vi "Recipe Editor.vi"() -> ()   [LabVIEW 2015, in "Formation.lvclass"]
uses:
  Formation.lvclass
  Type Defs/Action Enum.ctl
  Type Defs/Direction Enum.ctl
  Type Defs/SB Type Defs.lvlib
panel:
  out "Recipe 2":T3(array[cluster])
  out "Recipe":T3(array[cluster])=[{"Options"=[]}, {"Options"=[]}, {"Options"=[{"X"=1, "Y"=0, "SignMatch"=0, "Action"=enum."Attack", "Direction"=enum."N", "Unit Idx"=252}, {"X"=1, "Y"=1, "SignMatch"=0, "Action"=enum."Wait", "Direction"=enum."E", "Unit Idx"=2}]}, {"Options"=[{"X"=1, "Y"=0, "SignMatch"=0, "Action"=enum."Attack", "Direction"=enum."N", "Unit Idx"=253}, {"X"=1, "Y"=1, "SignMatch"=0, "Action"=enum."Wait", "Direction"=enum."E", "Unit Idx"=3}]}, {"Options"=[]}, {"Options"=[]}, {"Options"=[]}, {"Options"=[{"X"=0, "Y"=0, "SignMatch"=0, "Action"=enum."Attack", "Direction"=enum."NW", "Unit Idx"=0}, {"X"=1, "Y"=0, "SignMatch"=0, "Action"=enum."Attack", "Direction"=enum."N", "Unit Idx"=1}, {"X"=0, "Y"=1, "SignMatch"=0, "Action"=enum."Attack", "Direction"=enum."W", "Unit Idx"=6}, {"X"=1, "Y"=1, "SignMatch"=1, "Action"=enum."Wait", "Direction"=enum."E", "Unit Idx"=7}]}, {"Options"=[{"X"=1, "Y"=0, "SignMatch"=0, "Action"=enum."Move", "Direction"=enum."N", "Unit Idx"=2}, {"X"=1, "Y"=1, "SignMatch"=1, "Action"=enum."Wait", "Direction"=enum."E", "Unit Idx"=8}]}, {"Options"=[{"X"=1, "Y"=0, "SignMatch"=0, "Action"=enum."Move", "Direction"=enum."N", "Unit Idx"=3}, {"X"=1, "Y"=1, "SignMatch"=1, "Action"=enum."Wait", "Direction"=enum."E", "Unit Idx"=9}]}, {"Options"=[{"X"=2, "Y"=0, "SignMatch"=0, "Action"=enum."Attack", "Direction"=enum."NE", "Unit Idx"=5}, {"X"=1, "Y"=0, "SignMatch"=0, "Action"=enum."Attack", "Direction"=enum."N", "Unit Idx"=4}, {"X"=2, "Y"=1, "SignMatch"=0, "Action"=enum."Attack", "Direction"=enum."E", "Unit Idx"=11}, {"X"=1, "Y"=1, "SignMatch"=1, "Action"=enum."Wait", "Direction"=enum."E", "Unit Idx"=10}]}, {"Options"=[]}, {"Options"=[{"X"=0, "Y"=1, "SignMatch"=0, "Action"=enum."Attack", "Direction"=enum."W", "Unit Idx"=11}, {"X"=1, "Y"=1, "SignMatch"=0, "Action"=enum."Wait", "Direction"=enum."E", "Unit Idx"=12}]}, {"Options"=[{"X"=0, "Y"=1, "SignMatch"=0, "Action"=enum."Move", "Direction"=enum."W", "Unit Idx"=12}, {"X"=1, "Y"=0, "SignMatch"=0, "Action"=enum."Move", "Direction"=enum."N", "Unit Idx"=7}, {"X"=1, "Y"=1, "SignMatch"=1, "Action"=enum."Wait", "Direction"=enum."E", "Unit Idx"=13}]}, {"Options"=[{"X"=2, "Y"=1, "SignMatch"=0, "Action"=enum."Replicate", "Direction"=enum."E", "Unit Idx"=15}, {"X"=1, "Y"=2, "SignMatch"=0, "Action"=enum."Replicate", "Direction"=enum."S", "Unit Idx"=20}, {"X"=1, "Y"=0, "SignMatch"=0, "Action"=enum."Replicate", "Direction"=enum."N", "Unit Idx"=8}, {"X"=0, "Y"=1, "SignMatch"=0, "Action"=enum."Replicate", "Direction"=enum."W", "Unit Idx"=13}, {"X"=1, "Y"=1, "SignMatch"=1, "Action"=enum."Wait", "Direction"=enum."E", "Unit Idx"=14}]}, {"Options"=[{"X"=1, "Y"=2, "SignMatch"=0, "Action"=enum."Replicate", "Direction"=enum."S", "Unit Idx"=21}, {"X"=1, "Y"=0, "SignMatch"=0, "Action"=enum."Replicate", "Direction"=enum."N", "Unit Idx"=9}, {"X"=2, "Y"=1, "SignMatch"=0, "Action"=enum."Replicate", "Direction"=enum."E", "Unit Idx"=16}, {"X"=1, "Y"=1, "SignMatch"=1, "Action"=enum."Wait", "Direction"=enum."E", "Unit Idx"=15}]}, {"Options"=[{"X"=2, "Y"=1, "SignMatch"=0, "Action"=enum."Move", "Direction"=enum."E", "Unit Idx"=17}, {"X"=1, "Y"=0, "SignMatch"=0, "Action"=enum."Move", "Direction"=enum."N", "Unit Idx"=10}, {"X"=1, "Y"=1, "SignMatch"=1, "Action"=enum."Wait", "Direction"=enum."E", "Unit Idx"=16}]}, {"Options"=[{"X"=2, "Y"=1, "SignMatch"=0, "Action"=enum."Attack", "Direction"=enum."E", "Unit Idx"=18}, {"X"=1, "Y"=1, "SignMatch"=0, "Action"=enum."Wait", "Direction"=enum."E", "Unit Idx"=17}]}, {"Options"=[{"X"=0, "Y"=1, "SignMatch"=0, "Action"=enum."Attack", "Direction"=enum."W", "Unit Idx"=17}, {"X"=1, "Y"=1, "SignMatch"=0, "Action"=enum."Wait", "Direction"=enum."E", "Unit Idx"=18}]}, {"Options"=[{"X"=0, "Y"=1, "SignMatch"=0, "Action"=enum."Move", "Direction"=enum."W", "Unit Idx"=18}, {"X"=1, "Y"=2, "SignMatch"=0, "Action"=enum."Move", "Direction"=enum."S", "Unit Idx"=25}, {"X"=1, "Y"=1, "SignMatch"=1, "Action"=enum."Wait", "Direction"=enum."E", "Unit Idx"=19}]}, {"Options"=[{"X"=1, "Y"=0, "SignMatch"=0, "Action"=enum."Replicate", "Direction"=enum."N", "Unit Idx"=14}, {"X"=1, "Y"=2, "SignMatch"=0, "Action"=enum."Replicate", "Direction"=enum."S", "Unit Idx"=26}, {"X"=0, "Y"=1, "SignMatch"=0, "Action"=enum."Replicate", "Direction"=enum."W", "Unit Idx"=19}, {"X"=1, "Y"=1, "SignMatch"=1, "Action"=enum."Wait", "Direction"=enum."E", "Unit Idx"=20}]}, {"Options"=[{"X"=1, "Y"=0, "SignMatch"=0, "Action"=enum."Replicate", "Direction"=enum."N", "Unit Idx"=15}, {"X"=1, "Y"=2, "SignMatch"=0, "Action"=enum."Replicate", "Direction"=enum."S", "Unit Idx"=27}, {"X"=2, "Y"=1, "SignMatch"=0, "Action"=enum."Replicate", "Direction"=enum."E", "Unit Idx"=22}, {"X"=1, "Y"=1, "SignMatch"=1, "Action"=enum."Wait", "Direction"=enum."E", "Unit Idx"=21}]}, {"Options"=[{"X"=2, "Y"=1, "SignMatch"=0, "Action"=enum."Move", "Direction"=enum."E", "Unit Idx"=23}, {"X"=1, "Y"=2, "SignMatch"=0, "Action"=enum."Move", "Direction"=enum."S", "Unit Idx"=28}, {"X"=1, "Y"=1, "SignMatch"=1, "Action"=enum."Wait", "Direction"=enum."E", "Unit Idx"=22}]}, {"Options"=[{"X"=2, "Y"=1, "SignMatch"=0, "Action"=enum."Attack", "Direction"=enum."E", "Unit Idx"=24}, {"X"=1, "Y"=1, "SignMatch"=0, "Action"=enum."Wait", "Direction"=enum."E", "Unit Idx"=23}]}, {"Options"=[]}, {"Options"=[{"X"=0, "Y"=2, "SignMatch"=0, "Action"=enum."Attack", "Direction"=enum."SW", "Unit Idx"=30}, {"X"=0, "Y"=1, "SignMatch"=0, "Action"=enum."Attack", "Direction"=enum."W", "Unit Idx"=24}, {"X"=1, "Y"=2, "SignMatch"=0, "Action"=enum."Attack", "Direction"=enum."S", "Unit Idx"=31}, {"X"=1, "Y"=1, "SignMatch"=1, "Action"=enum."Wait", "Direction"=enum."E", "Unit Idx"=25}]}, {"Options"=[{"X"=1, "Y"=2, "SignMatch"=0, "Action"=enum."Move", "Direction"=enum."S", "Unit Idx"=32}, {"X"=1, "Y"=1, "SignMatch"=1, "Action"=enum."Wait", "Direction"=enum."E", "Unit Idx"=26}]}, {"Options"=[{"X"=1, "Y"=2, "SignMatch"=0, "Action"=enum."Move", "Direction"=enum."S", "Unit Idx"=33}, {"X"=1, "Y"=1, "SignMatch"=1, "Action"=enum."Wait", "Direction"=enum."E", "Unit Idx"=27}]}, {"Options"=[{"X"=2, "Y"=2, "SignMatch"=0, "Action"=enum."Attack", "Direction"=enum."SE", "Unit Idx"=35}, {"X"=1, "Y"=2, "SignMatch"=0, "Action"=enum."Attack", "Direction"=enum."S", "Unit Idx"=34}, {"X"=2, "Y"=1, "SignMatch"=0, "Action"=enum."Attack", "Direction"=enum."E", "Unit Idx"=29}, {"X"=1, "Y"=1, "SignMatch"=1, "Action"=enum."Wait", "Direction"=enum."E", "Unit Idx"=28}]}, {"Options"=[]}, {"Options"=[]}, {"Options"=[]}, {"Options"=[{"X"=1, "Y"=2, "SignMatch"=0, "Action"=enum."Attack", "Direction"=enum."S", "Unit Idx"=38}, {"X"=1, "Y"=1, "SignMatch"=0, "Action"=enum."Wait", "Direction"=enum."E", "Unit Idx"=32}]}, {"Options"=[{"X"=1, "Y"=2, "SignMatch"=0, "Action"=enum."Attack", "Direction"=enum."S", "Unit Idx"=39}, {"X"=1, "Y"=1, "SignMatch"=0, "Action"=enum."Wait", "Direction"=enum."E", "Unit Idx"=33}]}, {"Options"=[]}, {"Options"=[]}]
  in  "Apply":bool
  in  "SignMatch":i8
  in  "Formation":bool[][](array[boolean])
  in  "Action":T1
  in  "Unit ID":i32
  in  "Options":T4(array[cluster])=[{"X"=0, "Y"=1, "SignMatch"=-1, "Action"=enum."Attack", "Direction"=enum."W", "Unit Idx"=0}, {"X"=0, "Y"=0, "SignMatch"=-1, "Action"=enum."Attack", "Direction"=enum."NW", "Unit Idx"=0}, {"X"=1, "Y"=0, "SignMatch"=-1, "Action"=enum."Attack", "Direction"=enum."N", "Unit Idx"=0}, {"X"=2, "Y"=0, "SignMatch"=-1, "Action"=enum."Attack", "Direction"=enum."NE", "Unit Idx"=0}, {"X"=1, "Y"=1, "SignMatch"=1, "Action"=enum."Attack", "Direction"=enum."N", "Unit Idx"=0}]
  in  "Move Selection":bool[][](array[boolean])
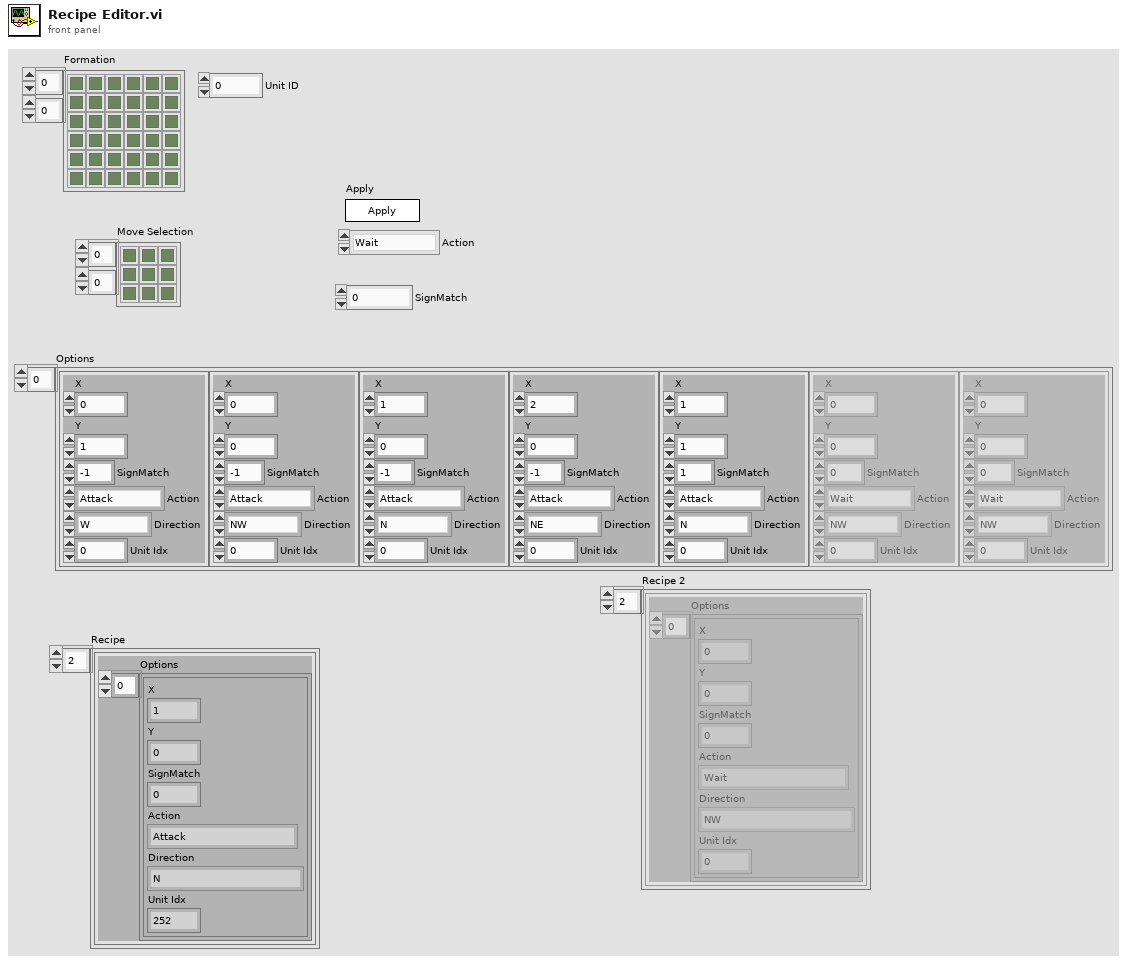
[diagram p1: front panel]
types:
  T1 = typedef "SB Type Defs.lvlib/Action Enum.ctl" = enum16{"Wait", "Move", "Attack", "Replicate"}
  T2 = typedef "SB Type Defs.lvlib/Direction Enum.ctl" = enum16{"NW", "N", "NE", "E", "SE", "S", "SW", "W"}
  T3 = cluster{"Options":cluster{"X":i8, "Y":i8, "SignMatch":i8, "Action":T1, "Direction":T2, "Unit Idx":u8}[]}[]
  T4 = cluster{"X":i8, "Y":i8, "SignMatch":i8, "Action":T1, "Direction":T2, "Unit Idx":u8}[]
  T5 = cluster{"Options":cluster{"X":i8, "Y":i8, "Sign":i8, "Action":T1, "Direction":T2, "Unit Idx":u8}[]}[]
  T6 = cluster{"X":i8, "Y":i8, "SignMatch":i8, "Action":T1, "Direction":T2, "Unit Idx":u8}
  T7 = cluster{cluster{"X":i8, "Y":i8, "SignMatch":i8, "Action":T1, "Direction":T2, "Unit Idx":u8}[]}
  T8 = cluster{"Options":cluster{"X":i8, "Y":i8, "SignMatch":i8, "Action":T1, "Direction":T2, "Unit Idx":u8}[]}
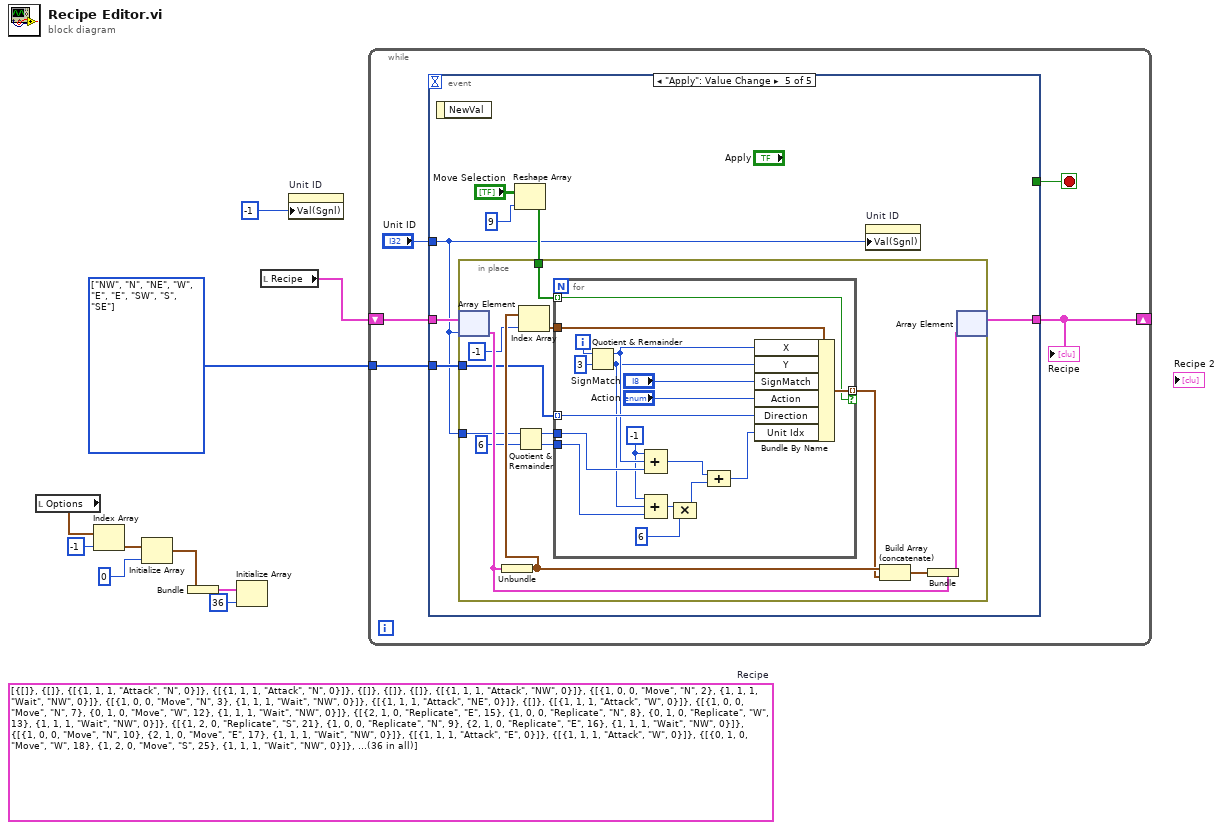
[diagram p0: block diagram]
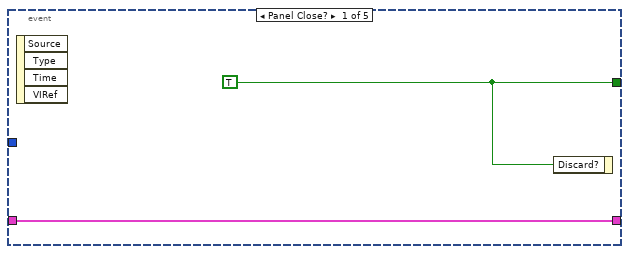
[diagram p2: hidden frame]
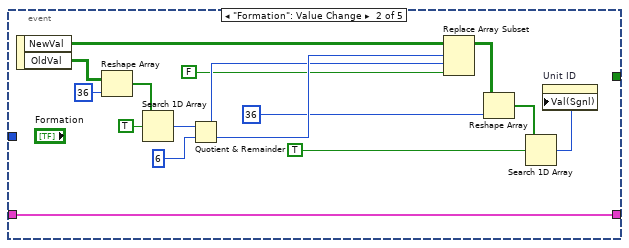
[diagram p3: hidden frame]
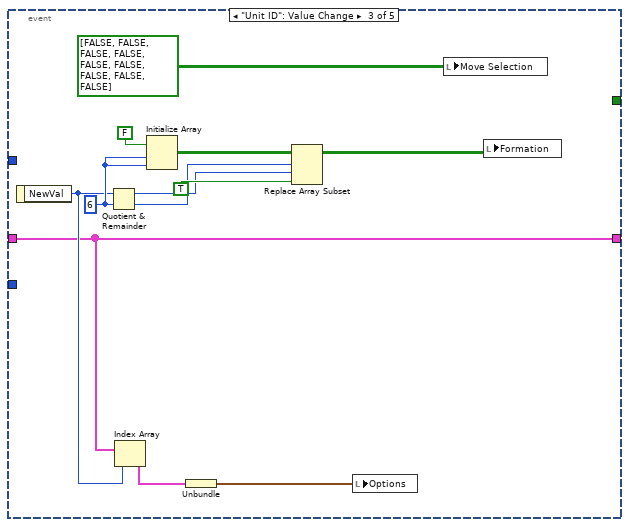
[diagram p4: hidden frame]
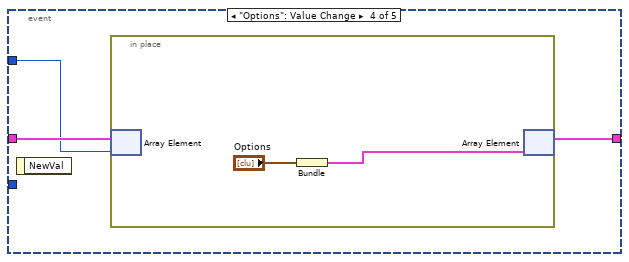
[diagram p5: hidden frame]
diagram:
  (unwired) T5 [{"Options"=[]}, {"Options"=[]}, {"Options"=[{"X"=1, "Y"=1, "Sign"=1, "Action"=enum."Attack", "Direction"=enum."N", "Unit Idx"=0}]}, {"Options"=[{"X"=1, "Y"=1, "Sign"=1, "Action"=enum."Attack", "Direction"=enum."N", "Unit Idx"=0}]}, {"Options"=[]}, {"Options"=[]}, {"Options"=[]}, {"Options"=[{"X"=1, "Y"=1, "Sign"=1, "Action"=enum."Attack", "Direction"=enum."NW", "Unit Idx"=0}]}, {"Options"=[{"X"=1, "Y"=0, "Sign"=0, "Action"=enum."Move", "Direction"=enum."N", "Unit Idx"=2}, {"X"=1, "Y"=1, "Sign"=1, "Action"=enum."Wait", "Direction"=enum."NW", "Unit Idx"=0}]}, {"Options"=[{"X"=1, "Y"=0, "Sign"=0, "Action"=enum."Move", "Direction"=enum."N", "Unit Idx"=3}, {"X"=1, "Y"=1, "Sign"=1, "Action"=enum."Wait", "Direction"=enum."NW", "Unit Idx"=0}]}, {"Options"=[{"X"=1, "Y"=1, "Sign"=1, "Action"=enum."Attack", "Direction"=enum."NE", "Unit Idx"=0}]}, {"Options"=[]}, {"Options"=[{"X"=1, "Y"=1, "Sign"=1, "Action"=enum."Attack", "Direction"=enum."W", "Unit Idx"=0}]}, {"Options"=[{"X"=1, "Y"=0, "Sign"=0, "Action"=enum."Move", "Direction"=enum."N", "Unit Idx"=7}, {"X"=0, "Y"=1, "Sign"=0, "Action"=enum."Move", "Direction"=enum."W", "Unit Idx"=12}, {"X"=1, "Y"=1, "Sign"=1, "Action"=enum."Wait", "Direction"=enum."NW", "Unit Idx"=0}]}, {"Options"=[{"X"=2, "Y"=1, "Sign"=0, "Action"=enum."Replicate", "Direction"=enum."E", "Unit Idx"=15}, {"X"=1, "Y"=0, "Sign"=0, "Action"=enum."Replicate", "Direction"=enum."N", "Unit Idx"=8}, {"X"=0, "Y"=1, "Sign"=0, "Action"=enum."Replicate", "Direction"=enum."W", "Unit Idx"=13}, {"X"=1, "Y"=1, "Sign"=1, "Action"=enum."Wait", "Direction"=enum."NW", "Unit Idx"=0}]}, {"Options"=[{"X"=1, "Y"=2, "Sign"=0, "Action"=enum."Replicate", "Direction"=enum."S", "Unit Idx"=21}, {"X"=1, "Y"=0, "Sign"=0, "Action"=enum."Replicate", "Direction"=enum."N", "Unit Idx"=9}, {"X"=2, "Y"=1, "Sign"=0, "Action"=enum."Replicate", "Direction"=enum."E", "Unit Idx"=16}, {"X"=1, "Y"=1, "Sign"=1, "Action"=enum."Wait", "Direction"=enum."NW", "Unit Idx"=0}]}, {"Options"=[{"X"=1, "Y"=0, "Sign"=0, "Action"=enum."Move", "Direction"=enum."N", "Unit Idx"=10}, {"X"=2, "Y"=1, "Sign"=0, "Action"=enum."Move", "Direction"=enum."E", "Unit Idx"=17}, {"X"=1, "Y"=1, "Sign"=1, "Action"=enum."Wait", "Direction"=enum."NW", "Unit Idx"=0}]}, {"Options"=[{"X"=1, "Y"=1, "Sign"=1, "Action"=enum."Attack", "Direction"=enum."E", "Unit Idx"=0}]}, {"Options"=[{"X"=1, "Y"=1, "Sign"=1, "Action"=enum."Attack", "Direction"=enum."W", "Unit Idx"=0}]}, {"Options"=[{"X"=0, "Y"=1, "Sign"=0, "Action"=enum."Move", "Direction"=enum."W", "Unit Idx"=18}, {"X"=1, "Y"=2, "Sign"=0, "Action"=enum."Move", "Direction"=enum."S", "Unit Idx"=25}, {"X"=1, "Y"=1, "Sign"=1, "Action"=enum."Wait", "Direction"=enum."NW", "Unit Idx"=0}]}, {"Options"=[{"X"=1, "Y"=0, "Sign"=0, "Action"=enum."Replicate", "Direction"=enum."N", "Unit Idx"=14}, {"X"=0, "Y"=1, "Sign"=0, "Action"=enum."Replicate", "Direction"=enum."W", "Unit Idx"=19}, {"X"=1, "Y"=2, "Sign"=0, "Action"=enum."Replicate", "Direction"=enum."S", "Unit Idx"=26}, {"X"=1, "Y"=1, "Sign"=1, "Action"=enum."Wait", "Direction"=enum."NW", "Unit Idx"=0}]}, {"Options"=[{"X"=0, "Y"=1, "Sign"=0, "Action"=enum."Replicate", "Direction"=enum."W", "Unit Idx"=15}, {"X"=2, "Y"=1, "Sign"=0, "Action"=enum."Replicate", "Direction"=enum."E", "Unit Idx"=22}, {"X"=1, "Y"=2, "Sign"=0, "Action"=enum."Replicate", "Direction"=enum."S", "Unit Idx"=27}, {"X"=1, "Y"=1, "Sign"=1, "Action"=enum."Wait", "Direction"=enum."NW", "Unit Idx"=0}]}, {"Options"=[{"X"=2, "Y"=1, "Sign"=0, "Action"=enum."Move", "Direction"=enum."E", "Unit Idx"=23}, {"X"=1, "Y"=2, "Sign"=0, "Action"=enum."Move", "Direction"=enum."S", "Unit Idx"=28}, {"X"=1, "Y"=1, "Sign"=1, "Action"=enum."Wait", "Direction"=enum."NW", "Unit Idx"=0}]}, {"Options"=[{"X"=1, "Y"=1, "Sign"=1, "Action"=enum."Attack", "Direction"=enum."E", "Unit Idx"=0}]}, {"Options"=[]}, {"Options"=[{"X"=1, "Y"=1, "Sign"=1, "Action"=enum."Attack", "Direction"=enum."SW", "Unit Idx"=0}]}, {"Options"=[{"X"=1, "Y"=2, "Sign"=0, "Action"=enum."Move", "Direction"=enum."S", "Unit Idx"=32}, {"X"=1, "Y"=1, "Sign"=1, "Action"=enum."Wait", "Direction"=enum."NW", "Unit Idx"=0}]}, {"Options"=[{"X"=1, "Y"=2, "Sign"=0, "Action"=enum."Move", "Direction"=enum."S", "Unit Idx"=33}, {"X"=1, "Y"=1, "Sign"=1, "Action"=enum."Wait", "Direction"=enum."NW", "Unit Idx"=0}]}, {"Options"=[{"X"=1, "Y"=1, "Sign"=1, "Action"=enum."Attack", "Direction"=enum."SE", "Unit Idx"=0}]}, {"Options"=[]}, {"Options"=[]}, {"Options"=[]}, {"Options"=[{"X"=1, "Y"=1, "Sign"=1, "Action"=enum."Attack", "Direction"=enum."S", "Unit Idx"=0}]}, {"Options"=[{"X"=1, "Y"=1, "Sign"=1, "Action"=enum."Attack", "Direction"=enum."S", "Unit Idx"=0}]}, {"Options"=[]}, {"Options"=[]}]  # Recipe
  w7 = T2[] [enum."NW", enum."N", enum."NE", enum."W", enum."E", enum."E", enum."SW", enum."S", enum."SE"] items=["NW", "N", "NE", "E", "SE", "S", "SW", "W"]
  n1 = local read "Options"() -> (w6:T4)
  n2 = Index Array(array=w6, index=-1) -> (element=w4:T6)
  n3 = Initialize Array(w4, 0 ("index")) -> (w2:T4)
  n4 = Bundle(w2) -> (w9:T7)  [unwired: 1 in]
  n5 = Initialize Array(w9, 36 ("dimension size")) -> ()  [unwired: 1 out]
  n6 = local read "Recipe"() -> (w1:T3)
  n7 = property on="Unit ID" class="DigNum (strict)"("Val(Sgnl)"=-1 ("index of element")) -> ()  [unwired: 2 in, 2 out]
  n8 = while {
    shift-right: [w12] -> _
    shift-left: w1 -> [w13]
    tunnel: w7 -> [w11]
    stop <- w15 stop-if-true
    n9 = event shown="[4] \"Apply\": Value Change" {
      selector: _ -> [_ _ _ _ _]
      dyn-events: _ -> [_ _ _ _ _]
      timeout: _ -> [_ _ _ _ _]
      tunnel: [w17 _ _ _ _] -> w15
      tunnel: "Unit ID" -> [_ _ _ w47 w51]
      tunnel: w13 -> [w16 w18 w36 w48 w57]
      tunnel: [w16 w18 w36 w46 w56] -> w12
      tunnel: w11 -> [_ _ _ _ w52]
      event Panel Close? {
        w17 = TRUE
        n10 = event-data() -> ()  [unwired: 1 in, 4 out]
        n11 = event-data("Discard?"=w17) -> ()  [unwired: 1 in, 1 out]
      }
      event "Formation": Value Change {
        n12 = event-data() -> ("NewVal"=w29:bool[][], "OldVal"=w33:bool[][])  [unwired: 1 in]
        n13 = Reshape Array(w33, 36 ("dimension size")) -> (w31:bool[])
        n14 = Search 1D Array(1D array=w31, element=TRUE) -> (index of element=w28:i32)  [unwired: 1 in]
        n15 = Quotient & Remainder(x=w28, y=6) -> (x-y*floor(x/y)=w25:i32, floor(x/y)=w26:i32)
        n16 = Replace Array Subset(array=w29, new element=FALSE ("new element/subarray"), index (row)=w26, index (col)=w25) -> (w22:bool[][])
        n17 = Reshape Array(w22, 36 ("dimension size")) -> (w20:bool[])
        n18 = Search 1D Array(1D array=w20, element=TRUE) -> (index of element=w19:i32)  [unwired: 1 in]
        n19 = property on="Unit ID" class="DigNum (strict)"("Val(Sgnl)"=w19) -> ()  [unwired: 2 in, 2 out]
      }
      event "Unit ID": Value Change {
        w44 = 6 ("y")
        n20 = event-data() -> ("NewVal"=w38:i32)  [unwired: 1 in]
        n21 = Quotient & Remainder(x=w38, y=w44) -> (x-y*floor(x/y)=w40:i32, floor(x/y)=w41:i32)
        n22 = Index Array(array=w36, index=w38) -> (element=w37:T8)
        n23 = Initialize Array(FALSE, w44, w44) -> (w43:bool[][])
        n24 = Unbundle(w37) -> ("Options"=w34:T4)
        n25 = Replace Array Subset(array=w43, new element=TRUE, index (row)=w41, index (col)=w40) -> (w39:bool[][])
        n26 = local write "Options"(w34) -> ()
        n27 = local write "Move Selection"(bool[][] [[FALSE, FALSE, FALSE], [FALSE, FALSE, FALSE], [FALSE, FALSE, FALSE]] ("Move Selection")) -> ()
        n28 = local write "Formation"(w39) -> ()
      }
      event "Options": Value Change {
        n29 = event-data() -> ()  [unwired: 1 in, 1 out]
        n30 = in-place {
          n31 = in-place-array #1(w48, w47) -> ()  [unwired: 1 out]
          n32 = Bundle("Options"="Options") -> (w49:T8)  [unwired: 1 in]
          n33 = in-place-array #1(w49) -> (w46:T3)  [unwired: 1 out]
        }
      }
      event "Apply": Value Change {
        n34 = event-data() -> ()  [unwired: 1 in, 1 out]
        n35 = Reshape Array("Move Selection", 9 ("dimension size")) -> (w53:bool[])
        n36 = in-place {
          in-place-border: w53 -> [w67]
          in-place-border: w52 -> [w62]
          in-place-border: w51 -> [w61]
          n37 = in-place-array #2(w57, w51) -> (w70:T8)
          n38 = Unbundle(w70) -> ("Options"=w66:T4)
          n39 = Quotient & Remainder(x=w61, y=6) -> (x-y*floor(x/y)=w59:i32, floor(x/y)=w58:i32)
          n40 = Index Array(array=w66, index=-1) -> (element=w64:T6)
          n41 = for {
            tunnel: w67 -> [w84] mode=indexing
            tunnel: w64 -> [w86]
            tunnel: [w85] -> w63 mode=indexing if=w84
            tunnel: w62 -> [w83] mode=indexing
            tunnel: w59 -> [w80]
            tunnel: w58 -> [w76]
            i -> [w88]
            w77 = -1 ("value")
            n42 = Quotient & Remainder(x=w88, y=3) -> (x-y*floor(x/y)=w79:i32, floor(x/y)=w78:i32)
            n43 = Compound Arithmetic op=ADD(w77, w79, w80) -> (w72:i32)
            n44 = Compound Arithmetic op=ADD(w77, w78, w76) -> (w75:i32)
            n45 = Compound Arithmetic op=MULTIPLY(w75, 6 ("value")) -> (w73:i32)
            n46 = Compound Arithmetic op=ADD(w72, w73) -> (w71:i32)
            n47 = Bundle By Name(cluster=w86, "X"=w79, "Y"=w78, "SignMatch"="SignMatch", "Action"="Action", "Direction"=w83, "Unit Idx"=w71) -> (w85:T6)
          }
          n48 = Build Array (concatenate)(w66, w63) -> (w68:T4)
          n49 = Bundle(cluster=w70, "Options"=w68) -> (w69:T8)
          n50 = in-place-array #2(w69) -> (w56:T3)  [unwired: 1 out]
        }
        n51 = property on="Unit ID" class="DigNum (strict)"("Val(Sgnl)"=w51) -> ()  [unwired: 2 in, 2 out]
      }
    }
    "Recipe" <- w12
  }
